vi "rwfm_CreateChan.vi"(8 "error in":errorcluster, 10 "Sensitivity":sgl[](array[numeric]), 11 "Dynamic FPGA VI Reference":T1) -> (0 "error out":errorcluster, 3 "Dynamic FPGA VI Reference":T1)   [LabVIEW 2017, in "cRIOWfmLib.lvlib"]
doc: "This VI collects and sends scaling coefficients as well as channel count to the FPGA. The number of elements in \"Channel Info\" must equal the number of channels acquired by the FPGA."
uses:
  <vilib>/addons/InsightCM/Devices/Shared/Cms/cRIOWfmAcq/cRIOWfmLib.lvlib
  <vilib>/addons/InsightCM/Devices/Shared/Cms/cRIOWfmAcq/subVIs/RIO Wfm Cust Ctrls/rwfm_DynamicFPGAref2.ctl
  <vilib>/Utility/error.llb/Error Cluster From Error Code.vi
  <vilib>/rvi/errors/niLvFpgaAdjustHostInterfaceError.vi
  <vilib>/rvi/interface/nirviReadWriteControl/nirviReadWriteControl.xnode
  <vilib>/rvi/interface/Simulation/niFpgaSimulationCallBeginRW.vi
  NiFpgaLv.dll
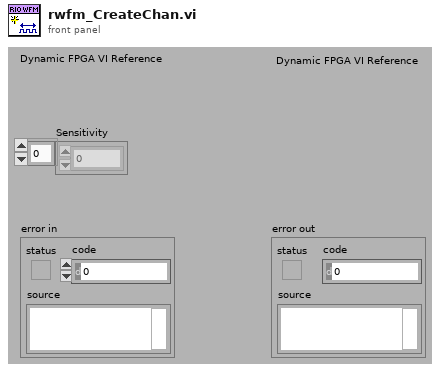
[diagram p1: front panel]
types:
  T1 = typedef "cRIOWfmLib.lvlib/rwfm_DynamicFPGAref2.ctl" = refnum<k20>
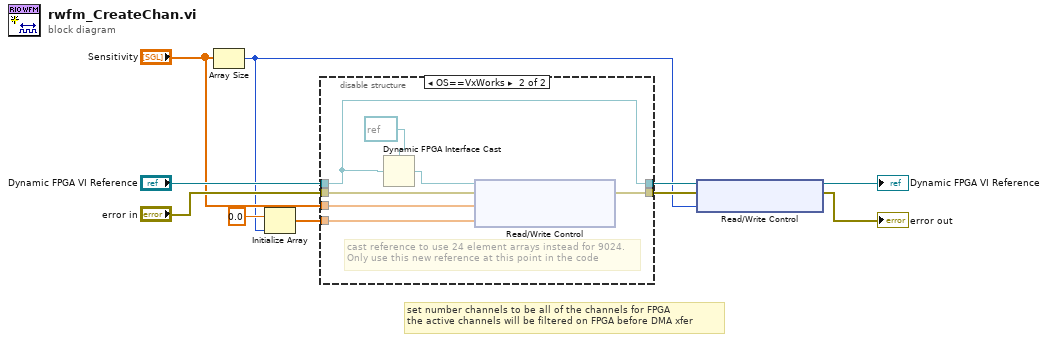
[diagram p0: block diagram]
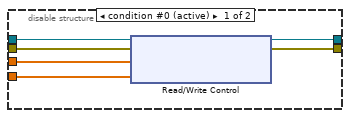
[diagram p2: hidden frame]
diagram:
  # "set number channels to be all of the channels for FPGA\nthe active channels will be filtered on FPGA before DMA xfer"
  n1 = Array Size(array="Sensitivity") -> (size(s)=w1:i32)
  n2 = Initialize Array(sgl 0.0, w1) -> (w4:sgl[])
  n3 = disable-structure shown="OS==VxWorks" {
    disable-tunnel: [w16 w19] -> w9
    disable-tunnel: [w15 w23] -> w8
    disable-tunnel: "error in" -> [w14 w22]
    disable-tunnel: "Dynamic FPGA VI Reference" -> [w13 w19]
    disable-tunnel: w4 -> [w12 w21]
    disable-tunnel: "Sensitivity" -> [w11 w20]
    frame condition #0 (active) {
      n4 = xnode "Read/Write Control"("FPGA VI Reference In"=w13, "error in"=w14, "Custom Scale Slope"=w11, "Custom Scale Intercept"=w12) -> ("FPGA VI Reference Out"=w16:T1, "error out"=w15:errorcluster)
    }
    frame condition #1 {
      # "cast reference to use 24 element arrays instead for 9024.\nOnly use this new reference at this point in the code"
      n5 = Dynamic FPGA Interface Cast(Session In=refnum<k20> refnum ("FPGA Interface"), Type=w19) -> (Session Out=w17:refnum<k20>)
      n6 = xnode "Read/Write Control"("FPGA VI Reference In"=w17, "error in"=w22, "Custom Scale Slope"=w20, "Custom Scale Intercept"=w21) -> ("error out"=w23:errorcluster)  [unwired: 1 out]
    }
  }
  n7 = xnode "Read/Write Control"("FPGA VI Reference In"=w9, "error in"=w8, "Total Avail Channels"=w1) -> ("FPGA VI Reference Out"=→"Dynamic FPGA VI Reference":T1, "error out"=→"error out":errorcluster)
